vi "GetText.vi"(8 "error in":errorcluster, 11 "Temperature Controller Logic editor node in":refnum<class "Temperature Controller Logic editor node.lvclass">) -> (0 "error out":errorcluster, 1 "additional text":string, 2 "text":string, 3 "Temperature Controller Logic editor node out":refnum<class "Temperature Controller Logic editor node.lvclass">, 4 "glyph":string)   [LabVIEW 2013, in "Temperature Controller Logic editor node.lvclass"]
uses:
  Temperature Controller Logic editor node.lvclass
  <vilib>/NI/Tag Bus Data Framework/Configuration Editor/PL Framework Configuration Tool.lvlib
  <vilib>/NI/Tag Bus Data Framework/fixed module parent/editor node/fixed channel editor.lvclass
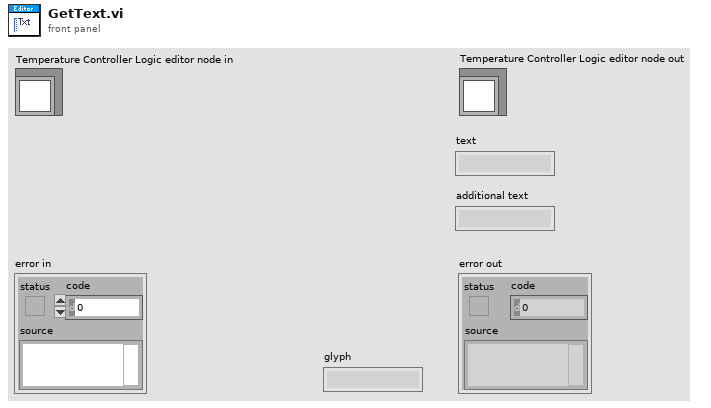
[diagram p1: front panel]
types:
  T1 = typedef "PL Framework Configuration Tool.lvlib/Glyphs Status.ctl" = enum16{"Normal", "Error", "Async"}
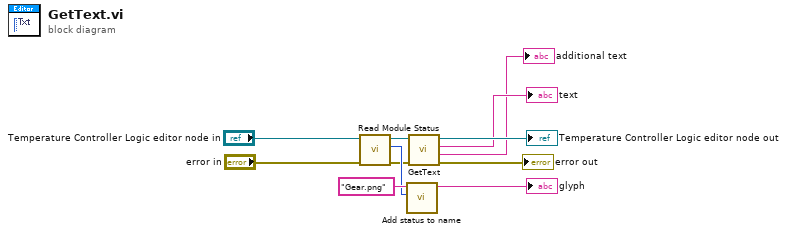
[diagram p0: block diagram]
diagram:
  n1 = call-dynamic "Read Module Status.vi"("error in"="error in", "Module Editor Node in"="Temperature Controller Logic editor node in") -> ("error out"=w8:errorcluster, "module status"=w10:T1, "Module Editor Node out"=w9:refnum<class "Temperature Controller Logic editor node.lvclass">)  [unwired: 7 in]
  n2 = call <vilib>:"Add status to name.vi"("Status"=w10, "Name"="Gear.png" ("glyph")) -> ("Name with status"=→"glyph":string)  [unwired: 9 in]
  n3 = call-parent "GetText.vi"("error in"=w8, "Module Editor Node in"=w9) -> ("error out"=→"error out":errorcluster, "additional text"=→"additional text":string, "text"=→"text":string, "Module Editor Node out"=→"Temperature Controller Logic editor node out":refnum<class "Temperature Controller Logic editor node.lvclass">)  [unwired: 5 in, 1 out]
